vi "Launcher.vi"   [LabVIEW 2024]
uses:
  Chef UI/Chef UI.lvclass
  <vilib>/ActorFramework/Actor/Actor.lvclass
  C:/Program Files/National Instruments/LabVIEW 2024/vi.lib/ActorFramework/Actor/Actor.lvclass
  C:/Users/burakkorkmaz/Desktop/PROJE/actor-state-machine/Chef UI/Chef UI.lvclass
  C:/Users/burakkorkmaz/Desktop/PROJE/actor-state-machine/Chef UI Logic/Chef UI Logic/Chef UI Logic.lvclass
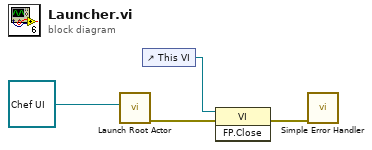
[diagram p0: block diagram]
diagram:
  n1 = call <vilib>:"Launch Root Actor.vi"("Actor"=refnum<class "Chef UI.lvclass"> refnum ("Chef UI.lvlib:Chef UI.lvclass")) -> ("error out"=w4:errorcluster)  [unwired: 9 in, 1 out]
  n2 = control-ref of="This VI"() -> (w3:refnum<vi>)
  n3 = invoke class="VI" method="FP.Close"(reference=w3, error in=w4) -> (error out=w2:errorcluster)  [unwired: 1 in, 2 out]
  n4 = call <vilib>:"Simple Error Handler.vi"("error in (no error)"=w2) -> ()  [unwired: 4 in, 5 out]
